vi "Initialize Sessions.vi"   [LabVIEW 2021, in "NI Session Management niSwitch.lvlib"]
uses:
  NI Session Management niSwitch.lvlib
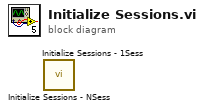
[diagram p0: block diagram]
diagram:
  n1 = call "Initialize Sessions - NSess.vi"() -> ()  [unwired: 8 in, 4 out]
  n2 = call "Initialize Sessions - 1Sess.vi"() -> ()  [unwired: 8 in, 4 out]
